vi "openOutFile.vi"(7 "Chemin de sortie":path, 8 "Entrée d'erreur":errorcluster caption="entrée d'erreur", 9 "Nom de l'analyse":string, 10 "Num de l'analyse":i32, 11 "VISA resource name":refnum<visa-resource-name>) -> (0 "Sortie d'erreur":errorcluster caption="sortie d'erreur", 1 "chaîne concaténée":string, 2 "refnum en sortie":refnum<file>, 3 "VISA resource name out":refnum<visa-resource-name>, 5 "chemin complet":path)   [LabVIEW 2019]
uses:
  <instrlib>/Sefram DAS240/Sefram DAS240.lvlib
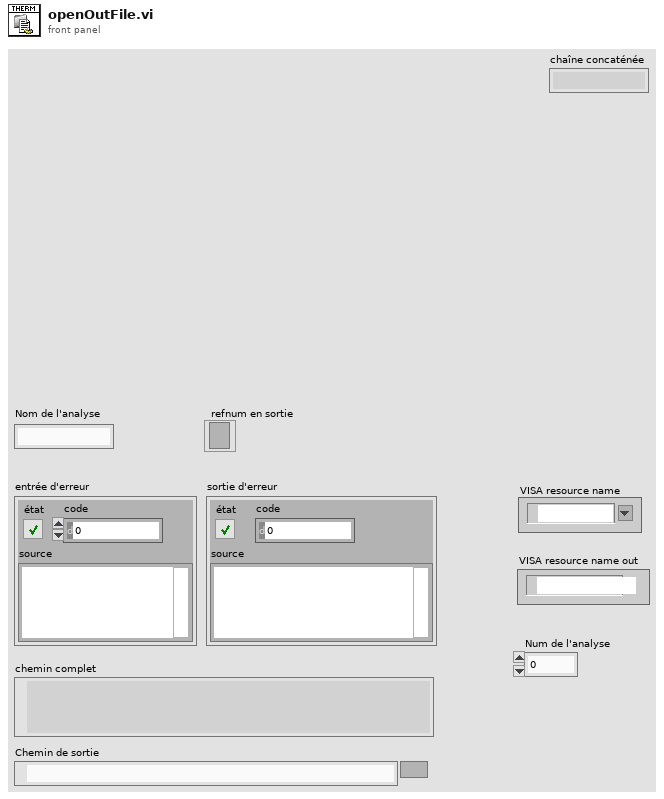
[diagram p1: front panel]
types:
  T1 = enum16{"open", "replace", "create", "open or create", "replace or create", "replace or create with confirmation"}
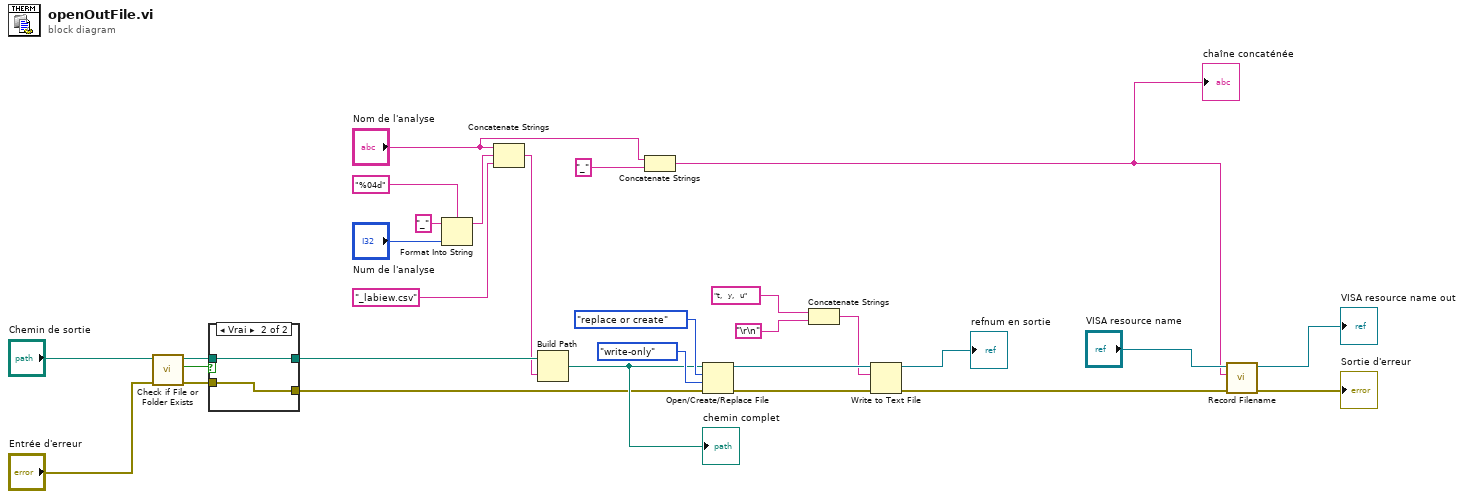
[diagram p0: block diagram]
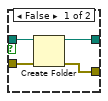
[diagram p2: hidden frame]
diagram:
  n1 = call <vilib>:"Check if File or Folder Exists.vi"("error in (no error)"="Entrée d'erreur", "path"="Chemin de sortie") -> ("error out"=w21:errorcluster, "file or folder exists?"=w23:bool, "dup path"=w22:path)  [unwired: 7 in]
  n2 = case shown="Vrai" w23 {
    tunnel: [w30 w35] -> w27
    tunnel: [w31 w34] -> w25
    tunnel: w22 -> [w33 w35]
    tunnel: w21 -> [w32 w34]
    frame False {
      n3 = Create Folder(path (use dialog)=w33, error in=w32) -> (created path=w30:path, error out=w31:errorcluster)  [unwired: 1 in, 1 out]
    }
    frame True {
    }
  }
  n4 = Format Into String(format string="%04d" ("chaîne de format"), initial string="_" ("chaîne initiale"), "Num de l'analyse") -> (resulting string=w6:string)  [unwired: 1 in, 1 out]
  n5 = Concatenate Strings("Nom de l'analyse", w6, "_labiew.csv" ("chaîne")) -> (w4:string)
  n6 = Build Path(base path=w27, name or relative path=w4) -> (appended path=w26:path)
  "chemin complet" <- w26
  n7 = Concatenate Strings("Nom de l'analyse", "_" ("chaîne")) -> (w1:string)
  "chaîne concaténée" <- w1
  n8 = Open/Create/Replace File(file path (use dialog)=w26, error in=w25, operation (0:open)=T1."replace or create" ("opération (0 : open)"), access (0:read/write)=enum16{"read/write", "read-only", "write-only"}."write-only" ("accès (0 : read/write)")) -> (refnum out=w18:refnum<file>, error out=w20:errorcluster)  [unwired: 2 in, 1 out]
  n9 = Concatenate Strings("t,   y,   u" ("texte"), "\r\n") -> (w15:string)
  n10 = Write to Text File(file (use dialog)=w18, text=w15, error in=w20) -> (refnum out=→"refnum en sortie":refnum<file>, error out=w12:errorcluster)  [unwired: 1 in, 1 out]
  n11 = call <instrlib>:"Record Filename.vi"("error in (no error)"=w12, "Filename"=w1, "VISA resource name"="VISA resource name") -> ("error out"=→"Sortie d'erreur":errorcluster, "VISA resource name out"=→"VISA resource name out":refnum<visa-resource-name>)  [unwired: 7 in]
